vi "SimpleGit_OnCommand(SingleObject).vi"(10 "Command ID":string, 11 "Object":T1) -> ()   [LabVIEW 2017]
uses:
  <resource>/Framework/Providers/API/ItemRef.ctl
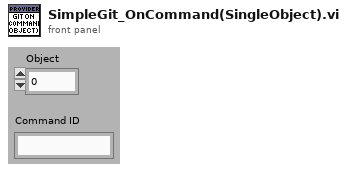
[diagram p1: front panel]
types:
  T1 = typedef "ItemRef.ctl" = u64
  T2 = enum16{"Action - None", "Action - RunPathInputVI"}
  T3 = enum16{"Action - None", "Action - RunPathInputVI", "Action - RunCmd", "Action - RunCmd with ProjPath"}
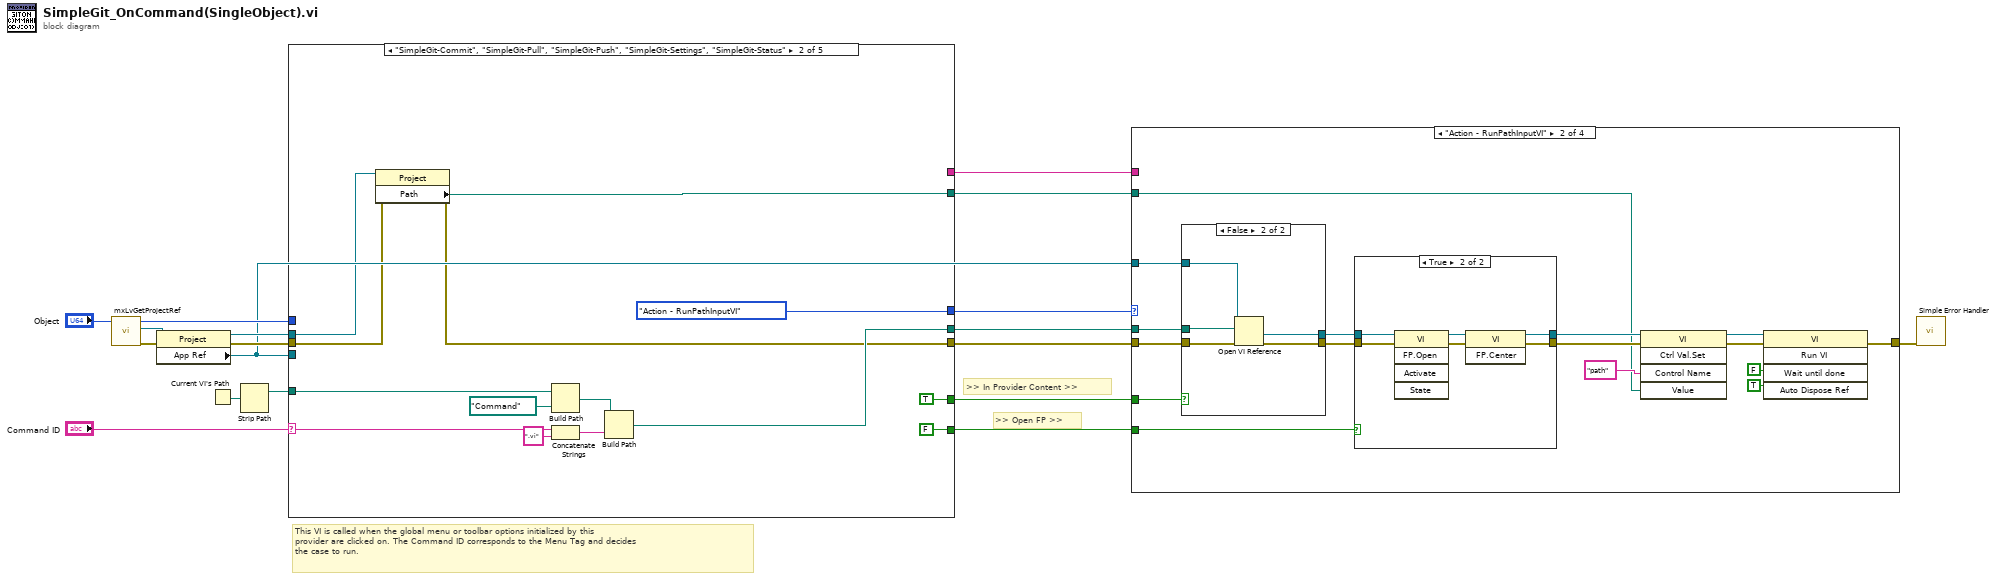
[diagram p0: block diagram]
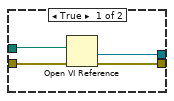
[diagram p4: hidden frame]
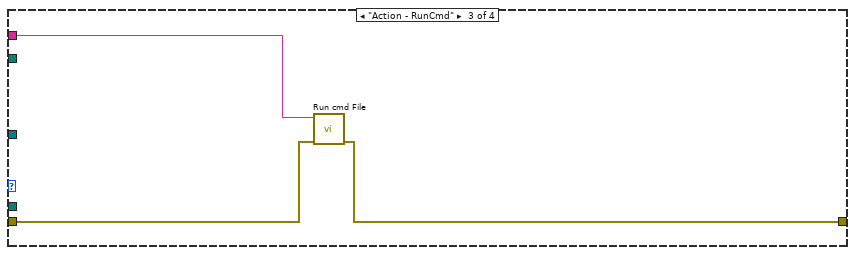
[diagram p5: hidden frame]
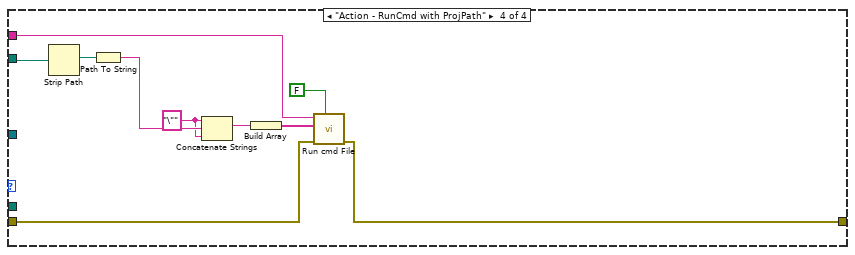
[diagram p6: hidden frame]
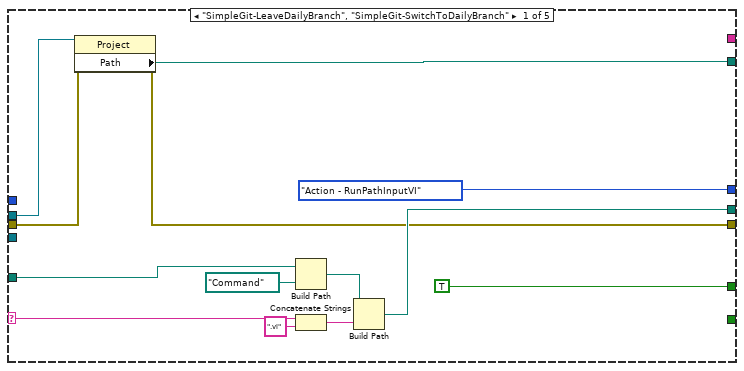
[diagram p7: hidden frame]
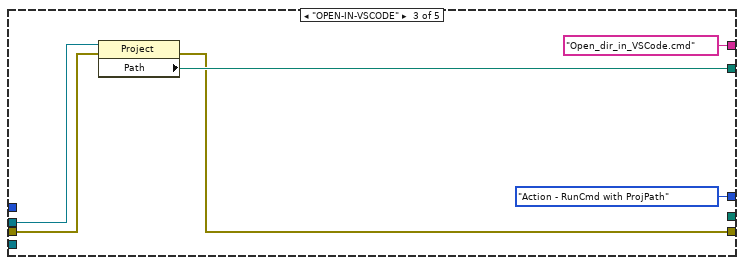
[diagram p8: hidden frame]
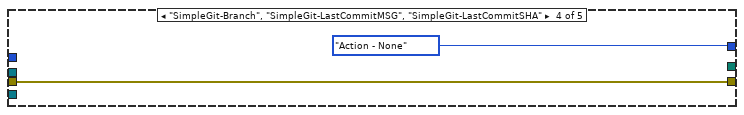
[diagram p9: hidden frame]
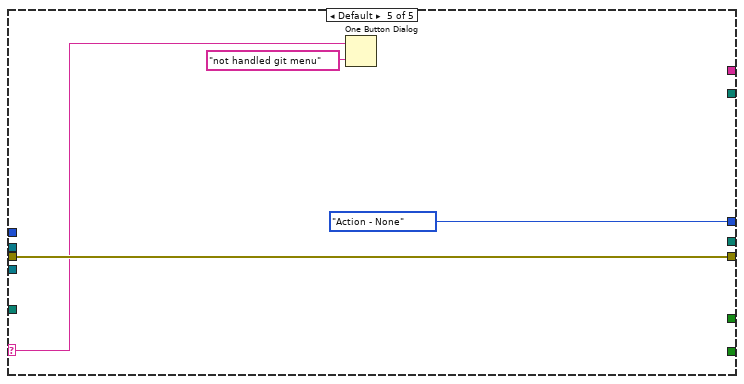
[diagram p10: hidden frame]
diagram:
  # ">> Open FP >>"
  # ">> In Provider Content >>"
  # "This VI is called when the global menu or toolbar options initialized by this \nprovider are clicked on. The Command ID corresponds to the Menu Tag and decides\nthe case to run."
  n1 = call <resource>:"mxLvGetProjectRef.vi"("Item"="Object") -> ("error out"=w17:errorcluster, "Project Refnum"=w16:refnum<vi>, "Item"=w14:T1)  [unwired: 8 in]
  n2 = property class="Project"(reference=w16, error in=w17) -> (reference out=w12:refnum<vi>, error out=w13:errorcluster, "App Ref"=w9:refnum<vi>)
  n3 = Current VI's Path() -> (path=w3:path)
  n4 = Strip Path(path=w3) -> (stripped path=w2:path)  [unwired: 1 out]
  n5 = case shown="\"SimpleGit-Commit\", \"SimpleGit-Pull\", \"SimpleGit-Push\", \"SimpleGit-Settings\", \"SimpleGit-Status\"" "Command ID" {
    selector: "Command ID" -> [w27 w39 _ _ w56]
    tunnel: [w22 w34 w46 w53 w57] -> w8
    tunnel: w14 -> [_ _ _ _ _]
    tunnel: w13 -> [w23 w35 w47 w53 w57]
    tunnel: w9 -> [_ _ _ _ _]
    tunnel: w12 -> [w24 w36 w49 _ _]
    tunnel: [T2."Action - RunPathInputVI" T2."Action - RunPathInputVI" T3."Action - RunCmd with ProjPath" T2."Action - None" T2."Action - None"] -> w10
    tunnel: [w28 w40 _ _ _] -> w7
    tunnel: [_ FALSE _ _ _] -> w6
    tunnel: [TRUE TRUE _ _ _] -> w5
    tunnel: [w21 w33 w48 _ _] -> w4
    tunnel: w2 -> [w19 w32 _ _ _]
    tunnel: [_ _ "Open_dir_in_VSCode.cmd" ("string") _ _] -> w1
    frame "SimpleGit-LeaveDailyBranch", "SimpleGit-SwitchToDailyBranch" {
      n6 = property class="Project"(reference=w24, error in=w23) -> (error out=w22:errorcluster, "Path"=w21:path)  [unwired: 1 out]
      n7 = Build Path(base path=w19, name or relative path=path "Command") -> (appended path=w29:path)
      n8 = Concatenate Strings(w27, ".vi" ("string")) -> (w25:string)
      n9 = Build Path(base path=w29, name or relative path=w25) -> (appended path=w28:path)
    }
    frame "SimpleGit-Commit", "SimpleGit-Pull", "SimpleGit-Push", "SimpleGit-Settings", "SimpleGit-Status" {
      n10 = property class="Project"(reference=w36, error in=w35) -> (error out=w34:errorcluster, "Path"=w33:path)  [unwired: 1 out]
      n11 = Build Path(base path=w32, name or relative path=path "Command") -> (appended path=w41:path)
      n12 = Concatenate Strings(w39, ".vi" ("string")) -> (w37:string)
      n13 = Build Path(base path=w41, name or relative path=w37) -> (appended path=w40:path)
    }
    frame "OPEN-IN-VSCODE" {
      n14 = property class="Project"(reference=w49, error in=w47) -> (error out=w46:errorcluster, "Path"=w48:path)  [unwired: 1 out]
    }
    frame "SimpleGit-Branch", "SimpleGit-LastCommitMSG", "SimpleGit-LastCommitSHA" {
    }
    frame Default {
      n15 = One Button Dialog(message=w56, button name ("OK")="not handled git menu") -> ()  [unwired: 1 out]
    }
  }
  n16 = case shown="\"Action - RunPathInputVI\"" w10 {
    tunnel: w8 -> [w58 w74 w92 w97]
    tunnel: w9 -> [_ w73 _ _]
    tunnel: [w58 w72 w93 w98] -> w11
    tunnel: w7 -> [_ w66 _ _]
    tunnel: w6 -> [_ w60 _ _]
    tunnel: w5 -> [_ w65 _ _]
    tunnel: w4 -> [_ w59 _ w104]
    tunnel: w1 -> [_ _ w94 w103]
    frame "Action - None", Default {
    }
    frame "Action - RunPathInputVI" {
      n17 = case shown="False" w65 {
        tunnel: w74 -> [w86 w91]
        tunnel: w73 -> [_ w90]
        tunnel: [w85 w89] -> w64
        tunnel: [w84 w88] -> w63
        tunnel: w66 -> [w83 w87]
        frame True {
          n18 = Open VI Reference(vi path=w83, error in (no error)=w86) -> (vi reference=w85:refnum<vi>, error out=w84:errorcluster)  [unwired: 4 in]
        }
        frame False {
          n19 = Open VI Reference(application reference (local)=w90, vi path=w87, error in (no error)=w91) -> (vi reference=w89:refnum<vi>, error out=w88:errorcluster)  [unwired: 3 in]
        }
      }
      n20 = case shown="True" w60 {
        tunnel: w64 -> [w76 w82]
        tunnel: [w76 w77] -> w61
        tunnel: [w75 w78] -> w62
        tunnel: w63 -> [w75 w81]
        frame False {
        }
        frame True {
          n21 = invoke class="VI" method="FP.Open"(reference=w82, error in=w81) -> (reference out=w80:refnum<vi>, error out=w79:errorcluster)  [unwired: 3 in, 3 out]
          n22 = invoke class="VI" method="FP.Center"(reference=w80, error in=w79) -> (reference out=w77:refnum<vi>, error out=w78:errorcluster)  [unwired: 1 in, 1 out]
        }
      }
      n23 = invoke class="VI" method="Ctrl Val.Set"(reference=w61, error in=w62, "Control Name"="path", "Value"=w59) -> (reference out=w68:refnum<vi>, error out=w67:errorcluster)  [unwired: 1 in, 3 out]
      n24 = invoke class="VI" method="Run VI"(reference=w68, error in=w67, "Wait until done"=FALSE ("Wait Until Done"), "Auto Dispose Ref"=TRUE ("Auto Dispose Reference")) -> (error out=w72:errorcluster)  [unwired: 1 in, 4 out]
    }
    frame "Action - RunCmd" {
      n25 = call "Run cmd File.vi"("Error in"=w92, "name or relative path"=w94) -> ("Error out"=w93:errorcluster)  [unwired: 7 in, 2 out]
    }
    frame "Action - RunCmd with ProjPath" {
      w100 = "\"" ("string")
      n26 = Strip Path(path=w104) -> (stripped path=w95:path)  [unwired: 1 out]
      n27 = Path To String(path=w95) -> (string=w102:string)
      n28 = Concatenate Strings(w100, w102, w100) -> (w101:string)
      n29 = Build Array(w101) -> (w99:string[])
      n30 = call "Run cmd File.vi"("wait until completion? (T)"=FALSE, "Error in"=w97, "args"=w99, "name or relative path"=w103) -> ("Error out"=w98:errorcluster)  [unwired: 5 in, 2 out]
    }
  }
  n31 = call <vilib>:"Simple Error Handler.vi"("error in (no error)"=w11) -> ()  [unwired: 4 in, 5 out]
